vi "Slope calculation.vi"() -> ()   [LabVIEW 2011]
doc: "Displays a standard dialog box that prompts users to enter information, such as a user name and password.\n--------------------\n\nThis Express VI is configured as follows:\n\nMessage to Display to the User:请输入用户名和密码，登录测试软件！\nThe inputs are: \nText Entry Box: UserName\nText Entry Box: Password"
uses:
  <vilib>/Analysis/NI_AALPro.lvlib
panel:
  out "Best Linear Fit":dbl[](array[numeric]) caption="最佳线性拟合"
  in  "X":dbl[](array[numeric])
  in  "Y":dbl[](array[numeric])
  in  "Cancel":bool
  in  "OK":bool caption="OK1"
  in  "Formula Factor":i32(listbox)=-1 caption="Spec_limit"
  # "IL Spec Calculation"
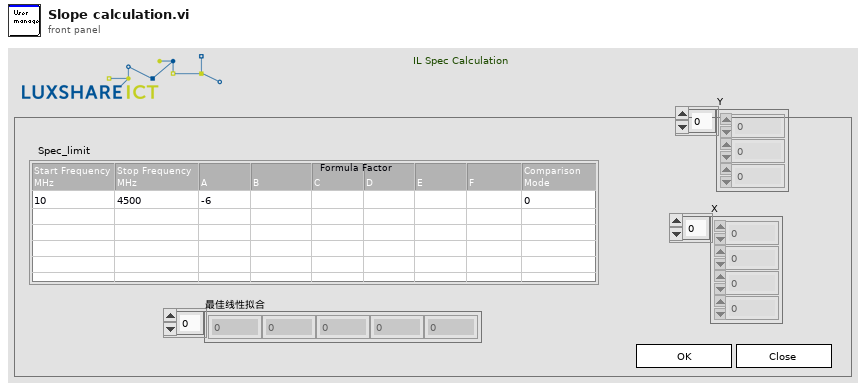
[diagram p1: front panel]
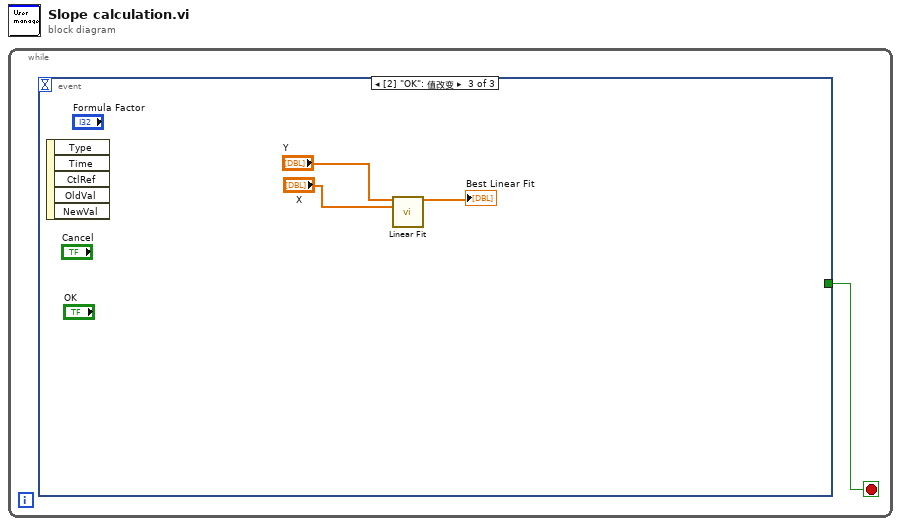
[diagram p0: block diagram]
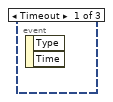
[diagram p2: hidden frame]
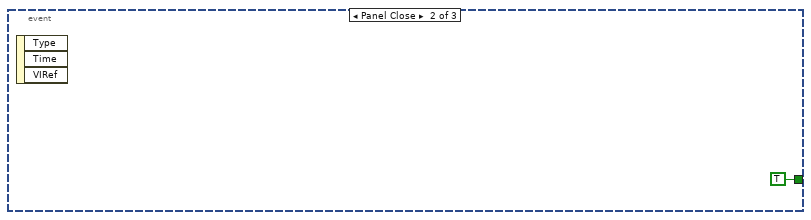
[diagram p3: hidden frame]
diagram:
  n1 = while {
    stop <- w1 stop-if-true
    n2 = event shown="[2] \"OK\": 值改变" {
      selector: _ -> [_ _ _]
      dyn-events: _ -> [_ _ _]
      timeout: _ -> [_ _ _]
      tunnel: [_ TRUE ("Cancel") _] -> w1
      event Timeout {
        n3 = event-data() -> ()  [unwired: 1 in, 2 out]
      }
      event Panel Close {
        n4 = event-data() -> ()  [unwired: 1 in, 3 out]
      }
      event "OK": Value Change {
        n5 = event-data() -> ()  [unwired: 1 in, 5 out]
        n6 = call <vilib>:"Linear Fit.vi"("Y"="Y", "X"="X") -> ("Best Linear Fit"=→"Best Linear Fit":dbl[])  [unwired: 9 in, 4 out]
      }
    }
  }
